vi "Report Error.vi"(8 "error in (no error)":errorcluster, 11 "EventLogHandler in":refnum<class "EventLogHandler.lvclass">) -> (0 "error out":errorcluster, 3 "EventLogHandler out":refnum<class "EventLogHandler.lvclass">)   [LabVIEW 2020, in "Vecto.lvlib" / "EventLogHandler.lvclass"]
uses:
  EventLogHandler.lvclass
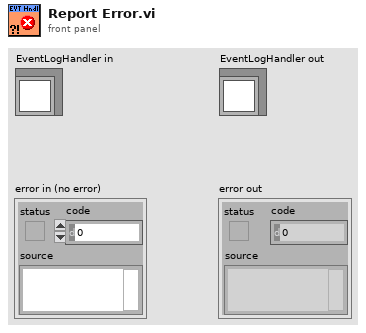
[diagram p1: front panel]
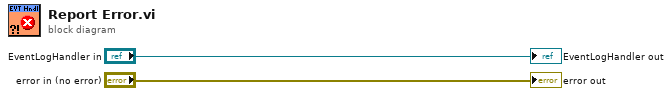
[diagram p0: block diagram]
diagram:
  "error out" <- "error in (no error)"
  "EventLogHandler out" <- "EventLogHandler in"
